vi "From Base Packet.vi"(8 "error in (no error)":errorcluster, 11 "Base Packet":refnum<class "Packet.lvclass">) -> (0 "error out":errorcluster, 3 "Literal out":refnum<class "Literal.lvclass">)   [LabVIEW 2020, in "Literal.lvclass"]
uses:
  Literal.lvclass
  C:/dev/IlluminatedG/AdventOfCode/2021/source/Day 16/Part 1/Packet/Packet.lvclass
  Packet/Packet.lvclass
  Literal.lvclass/Literal.ctl
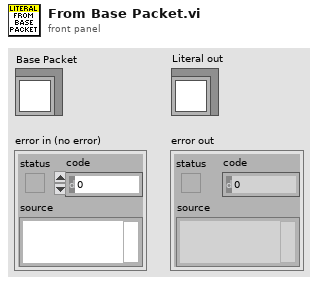
[diagram p1: front panel]
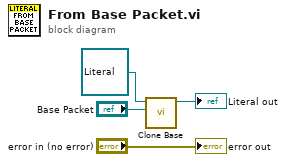
[diagram p0: block diagram]
diagram:
  n1 = call "Clone Base.vi"("From"="Base Packet", "Packet in"=refnum<class "Literal.lvclass"> refnum ("Literal.lvclass")) -> ("Packet out"=→"Literal out":refnum<class "Literal.lvclass">)  [unwired: 8 in, 1 out]
  "error out" <- "error in (no error)"
